vi "SVFA Peak Amplitude and Relative Phase (Nx1).vi"(0 "reference signal X":waveform(dbl), 1 "response signals Y [EUy]":waveform(dbl)[](array[waveform]), 2 "window":T9=1 items=["None"=0, "Hanning"=1, "Hamming"=2, "Blackman-Harris"=3, "Exact Blackman"=4, "Blackman"=5, "Flat Top"=6, "4 Term B-Harris "=7, "7 Term B-Harris"=8, "Low Sidelobe"=9, "Force - Exponential"=10, "Exponential"=65, "Blackman Nuttall"=11, "Triangle"=30, "Bartlett-Hanning"=31, "Bohman"=32, "Parzen"=33, "Welch"=34, "Kaiser"=60, "Dolph-Chebyshev"=61, "Gaussian"=62], 4 "view":T8={"dB On (T)"=FALSE, "unwrap phase (F)"=FALSE, "convert to degree (T)"=TRUE}, 5 "error in (no error)":errorcluster, 7 "averaging parameters":T7={"averaging mode"=enum."No averaging", "weighting mode"=enum."Exponential", "number of averages"=10, "linear mode"=enum."One shot"}, 8 "force and exponential window settings":cluster{"force [%]":dbl, "exponential [%]":dbl}={"force [%]"=50.0, "exponential [%]"=10.0} {"exponential [%]" min=0.0 max=100.0 format="%.2f"; "force [%]" min=0.0 max=100.0 format="%.2f"}, 9 "restart averaging (F)":bool) -> (11 "averaging done":bool, 12 "coherence":cluster{"f0":dbl, "df":dbl, "coherence":dbl[]}[](array[cluster]) {"coherence" format="%.2f"; "df" format="%.2f"; "f0" format="%.2f"}, 13 "averages completed":dbl, 14 "magnitudes [EUy pk]":cluster{"f0":dbl, "df":dbl, "magnitude":dbl[]}[](array[cluster]) {"magnitude" format="%.2p"; "df" format="%.2p"; "f0" format="%.2p"}, 15 "magnitude unit labels":string[](array[string]), 16 "phases":cluster{"f0":dbl, "df":dbl, "phase":dbl[]}[](array[cluster]) {"phase" format="%.2f"; "df" format="%.2f"; "f0" format="%.2f"}, 17 "phase unit labels":string[](array[string]), 18 "spectra info":T1[](array[typedef]) {"x-axis units" items=["Time (s)"=0, "Frequency-CB (Hz)"=1, "Frequency-CPB (Hz)"=1248, "Frequency-Arbitrary (Hz)"=2357, "Quefrency (s)"=2, "Revolutions (rev)"=3, "Order"=4, "Speed (RPM)"=11, "Speed (rad/s)"=21, "Index"=65535]; "weighting filter" items=["Linear", "A-weighting", "B-weighting", "C-weighting", "ITU-R 468-4", "Dolby", "CCITT", "C-message", "Wb", "Wc", "Wd", "We", "Wf", "Wh", "Wj", "Wk", "Wm", "AES17 20 kHz lowpass", "AES17 40 kHz lowpass", "AES17 20 kHz highpass", "AES17 40 kHz highpass"]; "dB reference [EU]" format="%.2f"; "engineering units" items=["custom..."=0, "V"=1, "A"=21, "C"=30, "pC"=31, "s"=32, "-"=29, "Pa"=2, "N"=20, "g"=3, "m/s^2"=4, "m/s"=5, "m"=6, "mm/s"=12, "mm"=13, "micron/s"=14, "micron"=15, "in/s^2"=7, "in/s"=8, "in"=9, "mil/s"=10, "mil"=11, "rad/s^2"=16, "rad/s"=17, "rad"=18, "deg/s^2"=26, "deg/s"=27, "deg"=28, "RPM"=22, "cycle/s^2"=23, "Hz"=24, "cycle"=25, "strain"=19]; "spectral info"."window" items=["None "=0, "Hanning"=1, "Hamming"=2, "Blackman-Harris"=3, "Exact Blackman"=4, "Blackman"=5, "Flat Top"=6, "4 Term B-Harris "=7, "7 Term B-Harris"=8, "Low Sidelobe"=9, "Force - Exponential"=10, "Gaussian"=62]}, 19 "error out":errorcluster)   [LabVIEW 2017]
doc: "Use this VI to compute FFT spectra with magnitude equal to response magnitude and phase equal to response relative to reference. Use the N responses, 1 stimulus instance to compute phase-assigned auto spectra for multiple response channels."
uses:
  <vilib>/addons/_NISVFA/_Shared subVIs/Controls/svc_Window [Dual FFT].ctl
  <vilib>/addons/_NISVFA/_Shared subVIs/Controls/svc_Spectrum Info.ctl
  <vilib>/addons/_NISVFA/_Shared subVIs/Controls/svc_X-Axis Units.ctl
  <vilib>/addons/_NISVFA/_Shared subVIs/Controls/svc_Spectrum Type.ctl
  <vilib>/addons/_NISVFA/_Shared subVIs/Controls/svc_Engineering Units Text Ring.ctl
  <vilib>/addons/_NISVFA/_Shared subVIs/Controls/svc_Weighting Filter Text Ring.ctl
  <vilib>/addons/_NISVFA/_Shared subVIs/Controls/svc_Complimentary Spectrum Units.ctl
  <vilib>/addons/_NISVFA/_Shared subVIs/Controls/svc_Window.ctl
  <vilib>/addons/_NISVFA/_Shared subVIs/Windowing/svfa_Scaled Time Domain Window (1 Ch).vi
  <vilib>/addons/_NISVFA/_Shared subVIs/Windowing/svfa_Scaled Time Domain Window (N Ch).vi
  <vilib>/addons/_NISVFA/_Shared subVIs/Windowing/svfa_Scaled Time Domain Window (Array).vi
  <vilib>/Analysis/4window.llb/Force Window.vi
  <vilib>/Analysis/4window.llb/Force Window (DBL).vi
  <vilib>/Analysis/4window.llb/Exponential Window.vi
  <vilib>/Analysis/4window.llb/Exponential Window (DBL).vi
  <vilib>/addons/_NISVFA/_Spectrum Processing/SVFA Unit Conversion (N Ch).vi
  <vilib>/addons/_NISVFA/_Baseband FFT/SVFA FFT Spectrum (Mag-Phase) (N Ch).vi
  <vilib>/addons/_NISVFA/_Baseband FFT/SVFA Frequency Response (Nx1) (Mag-Phase).vi
  <vilib>/Utility/error.llb/Error Cluster From Error Code.vi
  <vilib>/Analysis/0measdsp.llb/Scaled Time Domain Window.vi
  <vilib>/Analysis/0measdsp.llb/Scaled Time Domain Window (DBL).vi
  <vilib>/addons/_NISVFA/_Spectrum Processing/subVIs/svfa_Spectrum Info Window to windowTd Type Def.vi
  <vilib>/addons/_NISVFA/_Shared subVIs/Common/svc_Window Parameters.vi
  <vilib>/addons/_NISVFA/_Shared subVIs/Common/svc_Get Window Info.vi
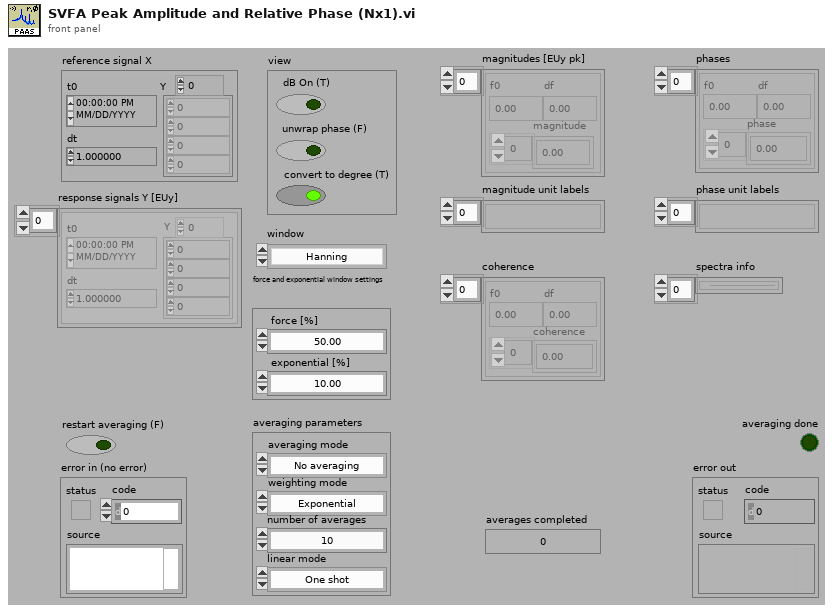
[diagram p1: front panel]
types:
  T1 = typedef "svc_Spectrum Info.ctl" = cluster{"channel name":string, "description":string, "x-axis units":T2, "spectral info":cluster{"spectrum type":T3, "linear/dB":enum16{"linear", "dB"}, "window":u16, "window size":i32, "FFT size":i32}, "engineering units":T4, "custom label":string, "dB reference [EU]":dbl, "peak units":enum16{"rms", "peak", "peak-peak"}, "weighting filter":T5, "spectral density?":bool, "unit label":string, "spectrum skewed?":bool, "complimentary spectrum units":T6}
  T2 = typedef "svc_X-Axis Units.ctl" = u16
  T3 = typedef "svc_Spectrum Type.ctl" = enum16{"FFT Spectrum [complex]", "Amplitude [Magnitude]", "Power [Magnitude^2]", "Cross Spectrum [complex]", "Frequency Response [Complex]"}
  T4 = typedef "svc_Engineering Units Text Ring.ctl" = u16
  T5 = typedef "svc_Weighting Filter Text Ring.ctl" = u16
  T6 = typedef "svc_Complimentary Spectrum Units.ctl" = enum16{"none", "radians", "degrees", "cycles", "imaginary"}
  T7 = cluster{"averaging mode":enum16{"No averaging", "Vector averaging", "RMS averaging", "Peak hold"}, "weighting mode":enum16{"Linear", "Exponential"}, "number of averages":u32, "linear mode":enum16{"One shot", "Auto restart"}}
  T8 = cluster{"dB On (T)":bool, "unwrap phase (F)":bool, "convert to degree (T)":bool}
  T9 = typedef "svc_Window [Dual FFT].ctl" = u32
  T10 = cluster{"linear/dB":enum16{"no change", "linear", "dB"}, "dB reference (0: no change)":dbl, "power/magnitude":enum16{"no change", "power", "magnitude"}, "view":enum16{"no change", "rms", "peak", "peak-peak"}}
  T11 = cluster{"dB On":bool, "unwrap phase":bool, "convert to degree":bool}
  T12 = typedef "svc_Window.ctl" = u32
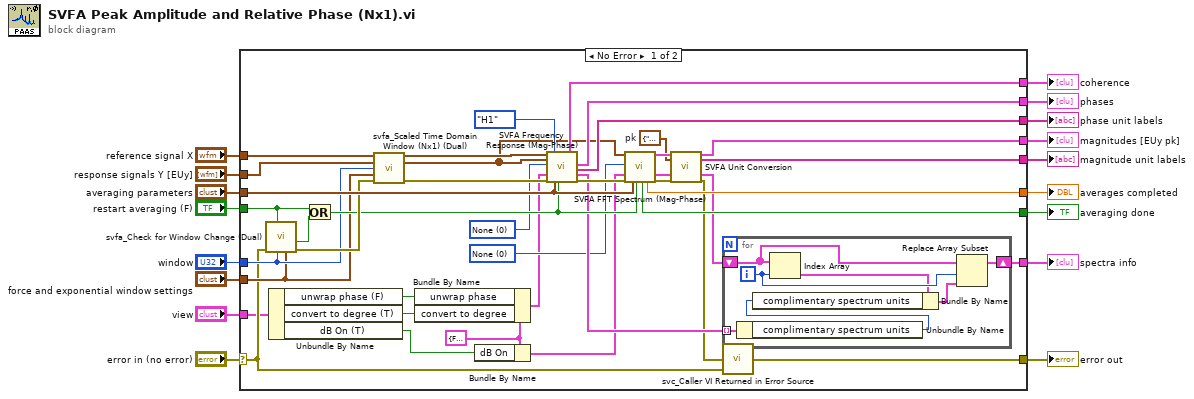
[diagram p0: block diagram]
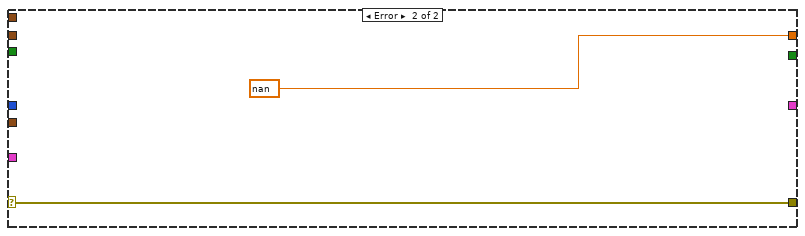
[diagram p2: hidden frame]
diagram:
  n1 = case shown="No Error" "error in (no error)" {
    selector: "error in (no error)" -> [w40 w66]
    tunnel: [w26 _] -> w17
    tunnel: [w56 _] -> w16
    tunnel: [w27 nan ("averages completed")] -> w15
    tunnel: [w55 _] -> w14
    tunnel: [w54 _] -> w13
    tunnel: [w38 _] -> w12
    tunnel: [w24 _] -> w11
    tunnel: [w23 _] -> w10
    tunnel: "view" -> [w34 _]
    tunnel: "averaging parameters" -> [w52 _]
    tunnel: "restart averaging (F)" -> [w49 _]
    tunnel: "window" -> [w47 _]
    tunnel: "force and exponential window settings" -> [w46 _]
    tunnel: "reference signal X" -> [w45 _]
    tunnel: "response signals Y [EUy]" -> [w43 _]
    tunnel: [w41 w66] -> w2
    frame No Error {
      w18 = T10 {"linear/dB"=enum."no change", "dB reference (0: no change)"=0.0, "power/magnitude"=enum."no change", "view"=enum."peak"}  # pk
      w36 = T11 {"dB On"=FALSE, "unwrap phase"=FALSE, "convert to degree"=FALSE} ("view")
      w37 = T12 0 items=["None"=0, "Hanning"=1, "Hamming"=2, "Blackman-Harris"=3, "Exact Blackman"=4, "Blackman"=5, "Flat Top"=6, "4 Term B-Harris "=7, "7 Term B-Harris"=8, "Low Sidelobe"=9, "Blackman Nuttall"=11, "Triangle"=30, "Bartlett-Hanning"=31, "Bohman"=32, "Parzen"=33, "Welch"=34, "Kaiser"=60, "Dolph-Chebyshev"=61, "Gaussian"=62] ("window")
      w29 = T9 0 items=["None"=0, "Hanning"=1, "Hamming"=2, "Blackman-Harris"=3, "Exact Blackman"=4, "Blackman"=5, "Flat Top"=6, "4 Term B-Harris "=7, "7 Term B-Harris"=8, "Low Sidelobe"=9, "Force - Exponential"=10, "Blackman Nuttall"=11, "Triangle"=30, "Bartlett-Hanning"=31, "Bohman"=32, "Parzen"=33, "Welch"=34, "Kaiser"=60, "Dolph-Chebyshev"=61, "Gaussian"=62] ("window")
      n2 = call <vilib>:"svfa_Check for Window Change (Dual).vi"("force/exp settings"=w46, "window"=w47, "restart averaging (F)"=w49, "error in (no error)"=w40) -> ("error out"=w51:errorcluster, "parameter has changed"=w50:bool)  [unwired: 6 in]
      n3 = Unbundle By Name(w34) -> ("unwrap phase (F)"=w32:bool, "convert to degree (T)"=w31:bool, "dB On (T)"=w30:bool)
      n4 = Or(x=w49, y=w50) -> (x .or. y?=w48:bool)
      n5 = call <vilib>:"svfa_Scaled Time Domain Window (Nx1) (Dual).vi"("stimulus signal X [EUx]"=w45, "response signals Y [EUy]"=w43, "window"=w47, "force and exponential window settings"=w46, "error in (no error)"=w51) -> ("stimulus signal X [EUx]"=w44:waveform(dbl), "response signals Y [EUy]"=w28:waveform(dbl)[], "error out"=w42:errorcluster)  [unwired: 6 in, 2 out]
      n6 = Bundle By Name(cluster=w36, "unwrap phase"=w32, "convert to degree"=w31) -> (w35:T11)
      n7 = Bundle By Name(cluster=w36, "dB On"=w30) -> (w33:T11)
      n8 = call-poly <vilib>:"SVFA Frequency Response (Mag-Phase).vi"("stimulus signal X [EUx]"=w44, "response signals Y [EUy]"=w28, "window"=w29, "view"=w35, "error in (no error)"=w42, "FRF mode"=enum16{"H1", "H2", "H3"}."H1", "averaging parameters"=w52, "restart averaging (F)"=w48) -> ("coherence"=w56:cluster{"f0":dbl, "df":dbl, "coherence":dbl[]}[], "phase [degrees]"=w55:cluster{"f0":dbl, "df":dbl, "phase":dbl[]}[], "phase unit labels"=w54:string[], "spectra info"=w39:T1[], "error out"=w53:errorcluster)  [unwired: 3 in, 4 out]
      n9 = call-poly <vilib>:"SVFA FFT Spectrum (Mag-Phase).vi"("scaled signals [EU]"=w28, "window"=w37, "view"=w33, "error in (no error)"=w53, "averaging parameters"=w52, "restart averaging (F)"=w48) -> ("averaging done"=w26:bool, "averages completed"=w27:dbl, "magnitudes [dB EU]"=w25:cluster{"f0":dbl, "df":dbl, "magnitude":dbl[]}[], "spectrum info"=w22:T1[], "error out"=w20:errorcluster)  [unwired: 6 in, 3 out]
      n10 = call-poly <vilib>:"SVFA Unit Conversion.vi"("spectra"=w25, "desired scaling"=w18, "spectrum info in"=w22, "error in (no error)"=w20) -> ("converted spectra"=w24:cluster{"x0":dbl, "dx":dbl, "magnitude":dbl[]}[], "unit labels"=w23:string[], "spectrum info out"=w21:T1[], "error out"=w19:errorcluster)  [unwired: 12 in]
      n11 = for {
        tunnel: w39 -> [w59] mode=indexing
        shift-right: [w63] -> w38
        shift-left: w21 -> [w64]
        i -> [w62]
        n12 = Unbundle By Name(w59) -> ("complimentary spectrum units"=w58:T6)
        n13 = Index Array(array=w64, index=w62) -> (element=w61:T1)
        n14 = Bundle By Name(cluster=w61, "complimentary spectrum units"=w58) -> (w60:T1)
        n15 = Replace Array Subset(array=w64, new element=w60, index=w62) -> (w63:T1[])
      }
      n16 = call <vilib>:"svc_Caller VI Returned in Error Source.vi"("warning input to caller"=w40, "error in (no error)"=w19) -> ("error out"=w41:errorcluster)  [unwired: 3 in]
    }
    frame Error {
    }
  }
  "averaging done" <- w17
  "coherence" <- w16
  "averages completed" <- w15
  "magnitudes [EUy pk]" <- w11
  "magnitude unit labels" <- w10
  "phases" <- w14
  "phase unit labels" <- w13
  "spectra info" <- w12
  "error out" <- w2
